vi "TR_Fill_listbox.vi"(8 "error in (no error)":errorcluster, 11 "Methods:TDMS files paths":path[](array[path])) -> (0 "error out":errorcluster, 2 "Listbox symbols IDs":i32[](array[numeric]), 3 "Listbox contents":string[][](array[string]))   [LabVIEW 2018, in "Tracks Repair.lvlib"]
uses:
  Tracks Repair.lvlib
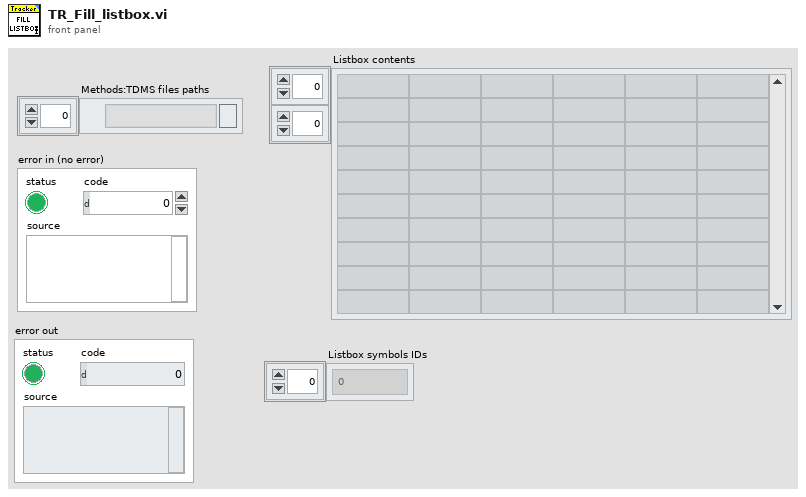
[diagram p1: front panel]
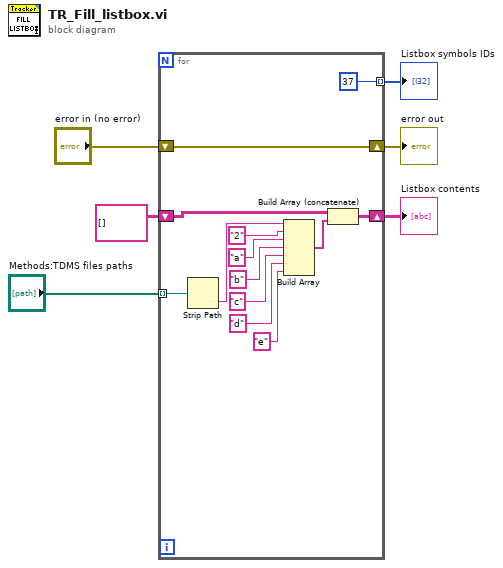
[diagram p0: block diagram]
diagram:
  n1 = for {
    tunnel: "Methods:TDMS files paths" -> [w18] mode=indexing
    shift-right: [w19] -> w5
    shift-left: "error in (no error)" -> [w19]
    shift-right: [w9] -> w2
    shift-left: string[][] [] -> [w11]
    tunnel: [37] -> w1 mode=indexing
    n2 = Strip Path(path=w18) -> (name=w17:string)  [unwired: 1 out]
    n3 = Build Array(w17, "2" ("element"), "a" ("element"), "b" ("element"), "c" ("element"), "d" ("element"), "e" ("element")) -> (w10:string[])
    n4 = Build Array (concatenate)(w11, w10) -> (w9:string[][])
  }
  "error out" <- w5
  "Listbox contents" <- w2
  "Listbox symbols IDs" <- w1
